vi "Identity Value.vi"(3 "Logger Identity in":refnum<class "Logger Identity.lvclass">) -> (1 "Value":string)   [LabVIEW 2020, in "VolatusData.lvlib" / "Logger Identity.lvclass"]
uses:
  Logger Identity.lvclass
  Logger Identity.lvclass/Logger Identity.ctl
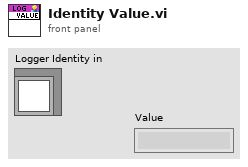
[diagram p1: front panel]
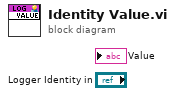
[diagram p0: block diagram]
diagram:
